vi "Teleop.vi"(10 "Match Info":T1={"Autonomous Elapsed Seconds"=0.0, "TeleOp Elapsed Seconds"=0.0, "Disabled Elapsed Seconds"=0.0, "Visited Autonomous"=FALSE, "Visited TeleOp"=FALSE, "Visited Disabled"=FALSE, "Autonomous Settings"={"Autonomous Style"=enum."Independent", "VI Refnum"=refnum}}, 11 "Call Context":T2) -> ()   [LabVIEW 2015]
doc: "This VI is called for each TeleOp packet received from the DS where the robot is not disabled. It is often used to read from the joysticks and update I/O or to update setpoints for timed control loops. It should complete and return within 20 milliseconds or it may miss DS packets."
uses:
  <vilib>/Rock Robotics/WPI/DriverStation/WPI_DriverStationDerivedRobotMode.ctl
  <vilib>/Rock Robotics/WPI/DriverStation/WPI_DriverStationMatch Info.ctl
  <vilib>/Rock Robotics/WPI/Utilities/WPI_GetSetVariantRefNum.vi
  Robot Global Data.vi
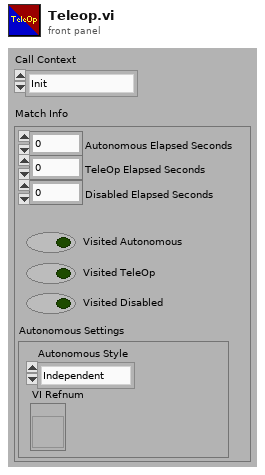
[diagram p1: front panel]
types:
  T1 = typedef "WPI_DriverStationMatch Info.ctl" = cluster{"Autonomous Elapsed Seconds":dbl, "TeleOp Elapsed Seconds":dbl, "Disabled Elapsed Seconds":dbl, "Visited Autonomous":bool, "Visited TeleOp":bool, "Visited Disabled":bool, "Autonomous Settings":cluster{"Autonomous Style":enum16{"Iterative", "Independent"}, "VI Refnum":refnum<vi>}}
  T2 = typedef "WPI_DriverStationDerivedRobotMode.ctl" = enum16{"Init", "Execute", "Stop"}
  T3 = typedef "WPI_JoystickDevRef.ctl" = cluster{"Device":T4}
  T4 = typedef "WPI_JoystickDeviceEnum.ctl" = enum16{"USB 0", "USB 1", "USB 2", "USB 3", "USB 4", "USB 5"}
  T5 = typedef "WPI_MotorControlDeviceRef.ctl" = cluster{"DeviceStatus":errorcluster, "Type":T6, "PWM":cluster{"PWM Channel":T7, "DeadBand":T8}, "CAN":cluster{"Device Number":u8, "Control Mode":T9, "Semaphore":T10, "Max Vout":dbl, "TalonSRX Control Mode":T11}, "Invert":bool}
  T6 = typedef "WPI_MotorControlType.ctl" = enum16{"PWM", "CAN", "CANTalonSRX"}
  T7 = typedef "FPGA_DIOPWMChannel.ctl" = enum8{"PWM 0", "PWM 1", "PWM 2", "PWM 3", "PWM 4", "PWM 5", "PWM 6", "PWM 7", "PWM 8", "PWM 9", "PWM MXP 0", "PWM MXP 1", "PWM MXP 2", "PWM MXP 3", "PWM MXP 4", "PWM MXP 5", "PWM MXP 6", "PWM MXP 7", "PWM MXP 8", "PWM MXP 9", "Invalid"}
  T8 = typedef "WPI_PWMDeadband.ctl" = cluster{"Name":string, "maxPositivePwm":i32, "minPositivePwm":i32, "centerPwm":i32, "maxNegativePwm":i32, "minNegativePwm":i32, "angularRange":u16}
  T9 = typedef "WPI_CANJaguar_ControlMode.ctl" = enum8{"Percent VBus", "Current", "Speed", "Position", "Voltage"}
  T10 = typedef "Semaphore RefNum" = refnum<k1>
  T11 = typedef "WPI_CANTalonSRX_APIControlMode.ctl" = enum8{"Percent VBus", "Speed", "Position", "Slave", "Unchanged / Invalid", "Voltage Compensation", "Current", "Motion Profile"}
  T12 = typedef "WPI_ServoDeviceRef.ctl" = cluster{"DeviceStatus":errorcluster, "PWM Channel":T7, "DeadBand":T8}
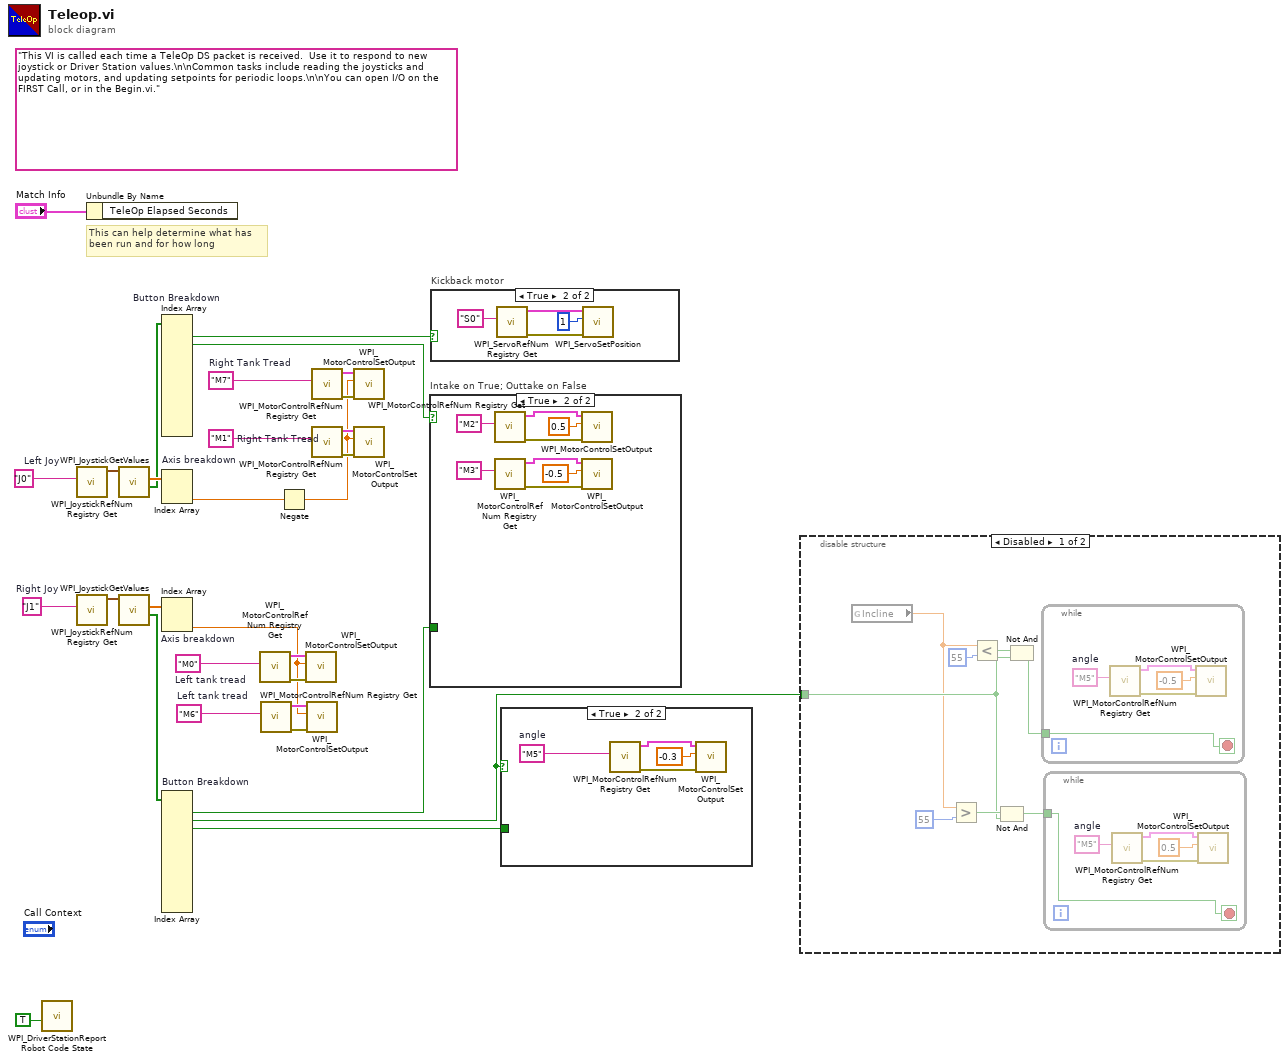
[diagram p0: block diagram]
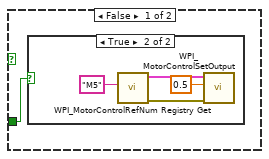
[diagram p3: hidden frame]
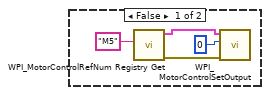
[diagram p4: hidden frame]
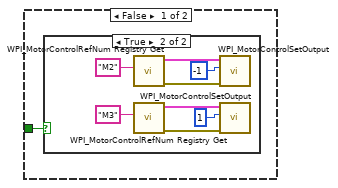
[diagram p5: hidden frame]
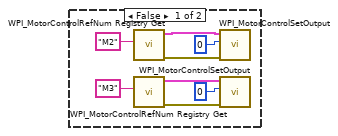
[diagram p6: hidden frame]
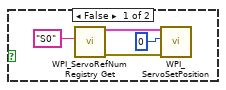
[diagram p7: hidden frame]
diagram:
  w8 = "M7"  # Right Tank Tread
  w10 = "M6"  # Left tank tread
  w16 = "M1"  # Right Tank Tread
  w18 = "M0"  # Left tank tread
  w24 = "J0"  # Left Joy
  (unwired) "This VI is called each time a TeleOp DS packet is received.  Use it to respond to new joystick or Driver Station values.\n\nCommon tasks include reading the joysticks and updating motors, and updating setpoints for periodic loops.\n\nYou can open I/O on the FIRST Call, or in the Begin.vi."
  w29 = "J1"  # Right Joy
  # "This can help determine what has\nbeen run and for how long"
  n1 = call <vilib>:"WPI_DriverStationReport Robot Code State.vi"("TeleOp"=TRUE ("Autonomous")) -> ()  [unwired: 10 in, 1 out]
  n2 = call <vilib>:"WPI_JoystickRefNum Registry Get.vi"("refnum name"=w24) -> ("JoystickDevRef"=w23:T3)  [unwired: 1 in, 9 out]
  n3 = call <vilib>:"WPI_JoystickRefNum Registry Get.vi"("refnum name"=w29) -> ("JoystickDevRef"=w28:T3)  [unwired: 1 in, 9 out]
  n4 = Unbundle By Name("Match Info") -> ()  [unwired: 1 out]
  n5 = call <vilib>:"WPI_JoystickGetValues.vi"("JoystickDevRef"=w23) -> ("Buttons"=w21:bool[], "Axes"=w22:dbl[])  [unwired: 6 in, 3 out]
  n6 = call <vilib>:"WPI_JoystickGetValues.vi"("JoystickDevRef"=w28) -> ("Buttons"=w25:bool[], "Axes"=w26:dbl[])  [unwired: 6 in, 3 out]
  n7 = Index Array "Button Breakdown"(array=w21) -> (element #1=w20:bool, element #2=w13:bool)  [unwired: 13 in, 11 out]
  n8 = Index Array "Axis breakdown"(array=w22) -> (element #2=w2:dbl)  [unwired: 2 in, 1 out]
  n9 = Index Array "Axis breakdown"(array=w26) -> (element #2=w3:dbl)  [unwired: 2 in, 1 out]
  n10 = Index Array "Button Breakdown"(array=w25) -> (element #1=w12:bool, element #2=w4:bool, element #3=w5:bool)  [unwired: 13 in, 10 out]
  n11 = call <vilib>:"WPI_MotorControlRefNum Registry Get.vi"("refnum name"=w18) -> ("error out"=w17:errorcluster, "MotorControlDevRef"=w19:T5)  [unwired: 9 in]
  n12 = call <vilib>:"WPI_MotorControlRefNum Registry Get.vi"("refnum name"=w10) -> ("error out"=w9:errorcluster, "MotorControlDevRef"=w11:T5)  [unwired: 9 in]
  n13 = Negate(x=w2) -> (-x=w1:dbl)
  n14 = call <vilib>:"WPI_MotorControlSetOutput.vi"("error in (no error)"=w17, "Output"=w3, "MotorControlDevRef"=w19) -> ()  [unwired: 6 in, 3 out]
  n15 = call <vilib>:"WPI_MotorControlSetOutput.vi"("error in (no error)"=w9, "Output"=w3, "MotorControlDevRef"=w11) -> ()  [unwired: 6 in, 3 out]
  n16 = call <vilib>:"WPI_MotorControlRefNum Registry Get.vi"("refnum name"=w8) -> ("error out"=w7:errorcluster, "MotorControlDevRef"=w6:T5)  [unwired: 9 in]
  n17 = call <vilib>:"WPI_MotorControlRefNum Registry Get.vi"("refnum name"=w16) -> ("error out"=w15:errorcluster, "MotorControlDevRef"=w14:T5)  [unwired: 9 in]
  n18 = call <vilib>:"WPI_MotorControlSetOutput.vi"("error in (no error)"=w7, "Output"=w1, "MotorControlDevRef"=w6) -> ()  [unwired: 6 in, 3 out]
  n19 = call <vilib>:"WPI_MotorControlSetOutput.vi"("error in (no error)"=w15, "Output"=w1, "MotorControlDevRef"=w14) -> ()  [unwired: 6 in, 3 out]
  n20 = case "Intake on True; Outtake on False" shown="True" w13 {
    tunnel: w12 -> [w31 _]
    frame False {
      n21 = case shown="True" w31 {
        frame False {
          n22 = call <vilib>:"WPI_MotorControlRefNum Registry Get.vi"("refnum name"="M2") -> ("error out"=w37:errorcluster, "MotorControlDevRef"=w38:T5)  [unwired: 9 in]
          n23 = call <vilib>:"WPI_MotorControlRefNum Registry Get.vi"("refnum name"="M3") -> ("error out"=w33:errorcluster, "MotorControlDevRef"=w34:T5)  [unwired: 9 in]
          n24 = call <vilib>:"WPI_MotorControlSetOutput.vi"("error in (no error)"=w37, "Output"=0, "MotorControlDevRef"=w38) -> ()  [unwired: 6 in, 3 out]
          n25 = call <vilib>:"WPI_MotorControlSetOutput.vi"("error in (no error)"=w33, "Output"=0, "MotorControlDevRef"=w34) -> ()  [unwired: 6 in, 3 out]
        }
        frame True {
          n26 = call <vilib>:"WPI_MotorControlRefNum Registry Get.vi"("refnum name"="M2") -> ("error out"=w45:errorcluster, "MotorControlDevRef"=w46:T5)  [unwired: 9 in]
          n27 = call <vilib>:"WPI_MotorControlRefNum Registry Get.vi"("refnum name"="M3") -> ("error out"=w41:errorcluster, "MotorControlDevRef"=w42:T5)  [unwired: 9 in]
          n28 = call <vilib>:"WPI_MotorControlSetOutput.vi"("error in (no error)"=w45, "Output"=-1, "MotorControlDevRef"=w46) -> ()  [unwired: 6 in, 3 out]
          n29 = call <vilib>:"WPI_MotorControlSetOutput.vi"("error in (no error)"=w41, "Output"=1, "MotorControlDevRef"=w42) -> ()  [unwired: 6 in, 3 out]
        }
      }
    }
    frame True {
      n30 = call <vilib>:"WPI_MotorControlRefNum Registry Get.vi"("refnum name"="M2") -> ("error out"=w53:errorcluster, "MotorControlDevRef"=w54:T5)  [unwired: 9 in]
      n31 = call <vilib>:"WPI_MotorControlRefNum Registry Get.vi"("refnum name"="M3") -> ("error out"=w49:errorcluster, "MotorControlDevRef"=w50:T5)  [unwired: 9 in]
      n32 = call <vilib>:"WPI_MotorControlSetOutput.vi"("error in (no error)"=w53, "Output"=0.5, "MotorControlDevRef"=w54) -> ()  [unwired: 6 in, 3 out]
      n33 = call <vilib>:"WPI_MotorControlSetOutput.vi"("error in (no error)"=w49, "Output"=-0.5, "MotorControlDevRef"=w50) -> ()  [unwired: 6 in, 3 out]
    }
  }
  n34 = case "Kickback motor" shown="True" w20 {
    frame False {
      n35 = call <vilib>:"WPI_ServoRefNum Registry Get.vi"("refnum name"="S0") -> ("error out"=w57:errorcluster, "ServoDeviceRef"=w58:T12)  [unwired: 9 in]
      n36 = call <vilib>:"WPI_ServoSetPosition.vi"("error in (no error)"=w57, "Position"=0, "ServoDeviceRef"=w58) -> ()  [unwired: 7 in, 2 out]
    }
    frame True {
      n37 = call <vilib>:"WPI_ServoRefNum Registry Get.vi"("refnum name"="S0") -> ("error out"=w61:errorcluster, "ServoDeviceRef"=w62:T12)  [unwired: 9 in]
      n38 = call <vilib>:"WPI_ServoSetPosition.vi"("error in (no error)"=w61, "Position"=1, "ServoDeviceRef"=w62) -> ()  [unwired: 7 in, 2 out]
    }
  }
  n39 = case shown="True" w4 {
    tunnel: w5 -> [w64 _]
    frame False {
      n40 = case "Intake on True; Outtake on False" shown="True" w64 {
        frame False {
          n41 = call <vilib>:"WPI_MotorControlRefNum Registry Get.vi"("refnum name"="M5") -> ("error out"=w66:errorcluster, "MotorControlDevRef"=w67:T5)  [unwired: 9 in]
          n42 = call <vilib>:"WPI_MotorControlSetOutput.vi"("error in (no error)"=w66, "Output"=0, "MotorControlDevRef"=w67) -> ()  [unwired: 6 in, 3 out]
        }
        frame True {
          n43 = call <vilib>:"WPI_MotorControlRefNum Registry Get.vi"("refnum name"="M5") -> ("error out"=w70:errorcluster, "MotorControlDevRef"=w71:T5)  [unwired: 9 in]
          n44 = call <vilib>:"WPI_MotorControlSetOutput.vi"("error in (no error)"=w70, "Output"=0.5, "MotorControlDevRef"=w71) -> ()  [unwired: 6 in, 3 out]
        }
      }
    }
    frame True {
      w75 = "M5"  # angle
      n45 = call <vilib>:"WPI_MotorControlRefNum Registry Get.vi"("refnum name"=w75) -> ("error out"=w74:errorcluster, "MotorControlDevRef"=w76:T5)  [unwired: 9 in]
      n46 = call <vilib>:"WPI_MotorControlSetOutput.vi"("error in (no error)"=w74, "Output"=-0.3, "MotorControlDevRef"=w76) -> ()  [unwired: 6 in, 3 out]
    }
  }
  n47 = disable-structure shown="Disabled" {
    disable-tunnel: w4 -> [w79 _]
    frame Disabled {
      n48 = global read "Robot Global Data.vi" "Incline"() -> (w77:dbl)
      n49 = Greater?(x=w77, y=55) -> (0:w81:bool)
      n50 = Less?(x=w77, y=55) -> (x < y?=w83:bool)
      n51 = Not And(1:w79, 2:w81) -> (0:w78:bool)
      n52 = Not And(1:w79, 2:w83) -> (0:w82:bool)
      n53 = while {
        tunnel: w82 -> [w90]
        stop <- w90 stop-if-true
        w93 = "M5"  # angle
        n54 = call <vilib>:"WPI_MotorControlRefNum Registry Get.vi"("refnum name"=w93) -> ("error out"=w92:errorcluster, "MotorControlDevRef"=w94:T5)  [unwired: 9 in]
        n55 = call <vilib>:"WPI_MotorControlSetOutput.vi"("error in (no error)"=w92, "Output"=-0.5, "MotorControlDevRef"=w94) -> ()  [unwired: 6 in, 3 out]
      }
      n56 = while {
        tunnel: w78 -> [w85]
        stop <- w85 stop-if-true
        w88 = "M5"  # angle
        n57 = call <vilib>:"WPI_MotorControlRefNum Registry Get.vi"("refnum name"=w88) -> ("error out"=w87:errorcluster, "MotorControlDevRef"=w89:T5)  [unwired: 9 in]
        n58 = call <vilib>:"WPI_MotorControlSetOutput.vi"("error in (no error)"=w87, "Output"=0.5, "MotorControlDevRef"=w89) -> ()  [unwired: 6 in, 3 out]
      }
    }
    frame Enabled {
    }
  }
